vi "Read Customer Name.vi"(11 "Abstract Beverage in":refnum<class "Abstract Beverage.lvclass">) -> (2 "Customer Name":string)   [LabVIEW 2013, in "Abstract Beverage.lvclass"]
uses:
  Abstract Beverage.lvclass
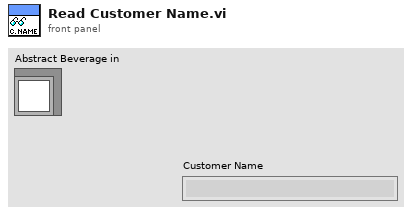
[diagram p1: front panel]
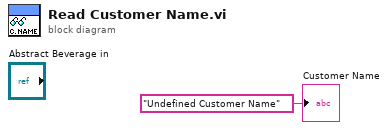
[diagram p0: block diagram]
diagram:
  "Customer Name" <- "Undefined Customer Name" ("Customer Name")
